vi "Leap Read.vi"(8 "error in (no error)":errorcluster, 11 "Leap Handle In":T14) -> (0 "error out":errorcluster, 2 "Frame":T1, 3 "Leap Handle Passthrough":T14, 5 "Leap Connected?":bool)   [LabVIEW 2011, in "LVH-Leap.lvlib"]
doc: "<b>Leap Read</b> requests and parses a <b>Frame</b> of data from the Leap Motion Controller. All the data associated with the Frame is organized into a LabVIEW cluster for accessibility.\n\nSpecifics about the data in the Frame cluster can be found by going to <b>Help » Leap Motion Controller Help</b> inside of LabVIEW"
uses:
  LVH-Leap.lvlib
  Private/Type Defs/Leap Handle.ctl
  C:/github/labviewhacker/LVH-Leap/LabVIEW/vi.lib/LabVIEW Hacker/Leap/Private/Libs/LeapCSharp.NET3.5.dll
  Private/Libs/LeapCSharp.NET3.5.dll
  Private/Type Defs/Frame.ctl
  Private/Type Defs/Hand.ctl
  Private/Type Defs/Vector.ctl
  Private/Type Defs/Pointable.ctl
  Private/Type Defs/Pointable Type.ctl
  Private/Type Defs/Pointable Zone.ctl
  Private/Type Defs/Gesture Key Tap.ctl
  Private/Type Defs/Gesture Common.ctl
  Private/Type Defs/Gesture Type.ctl
  Private/Type Defs/Gesture State.ctl
  Private/Type Defs/Gesture Screen Tap.ctl
  Private/Type Defs/Gesture Circle.ctl
  Private/Type Defs/Gesture Swipe.ctl
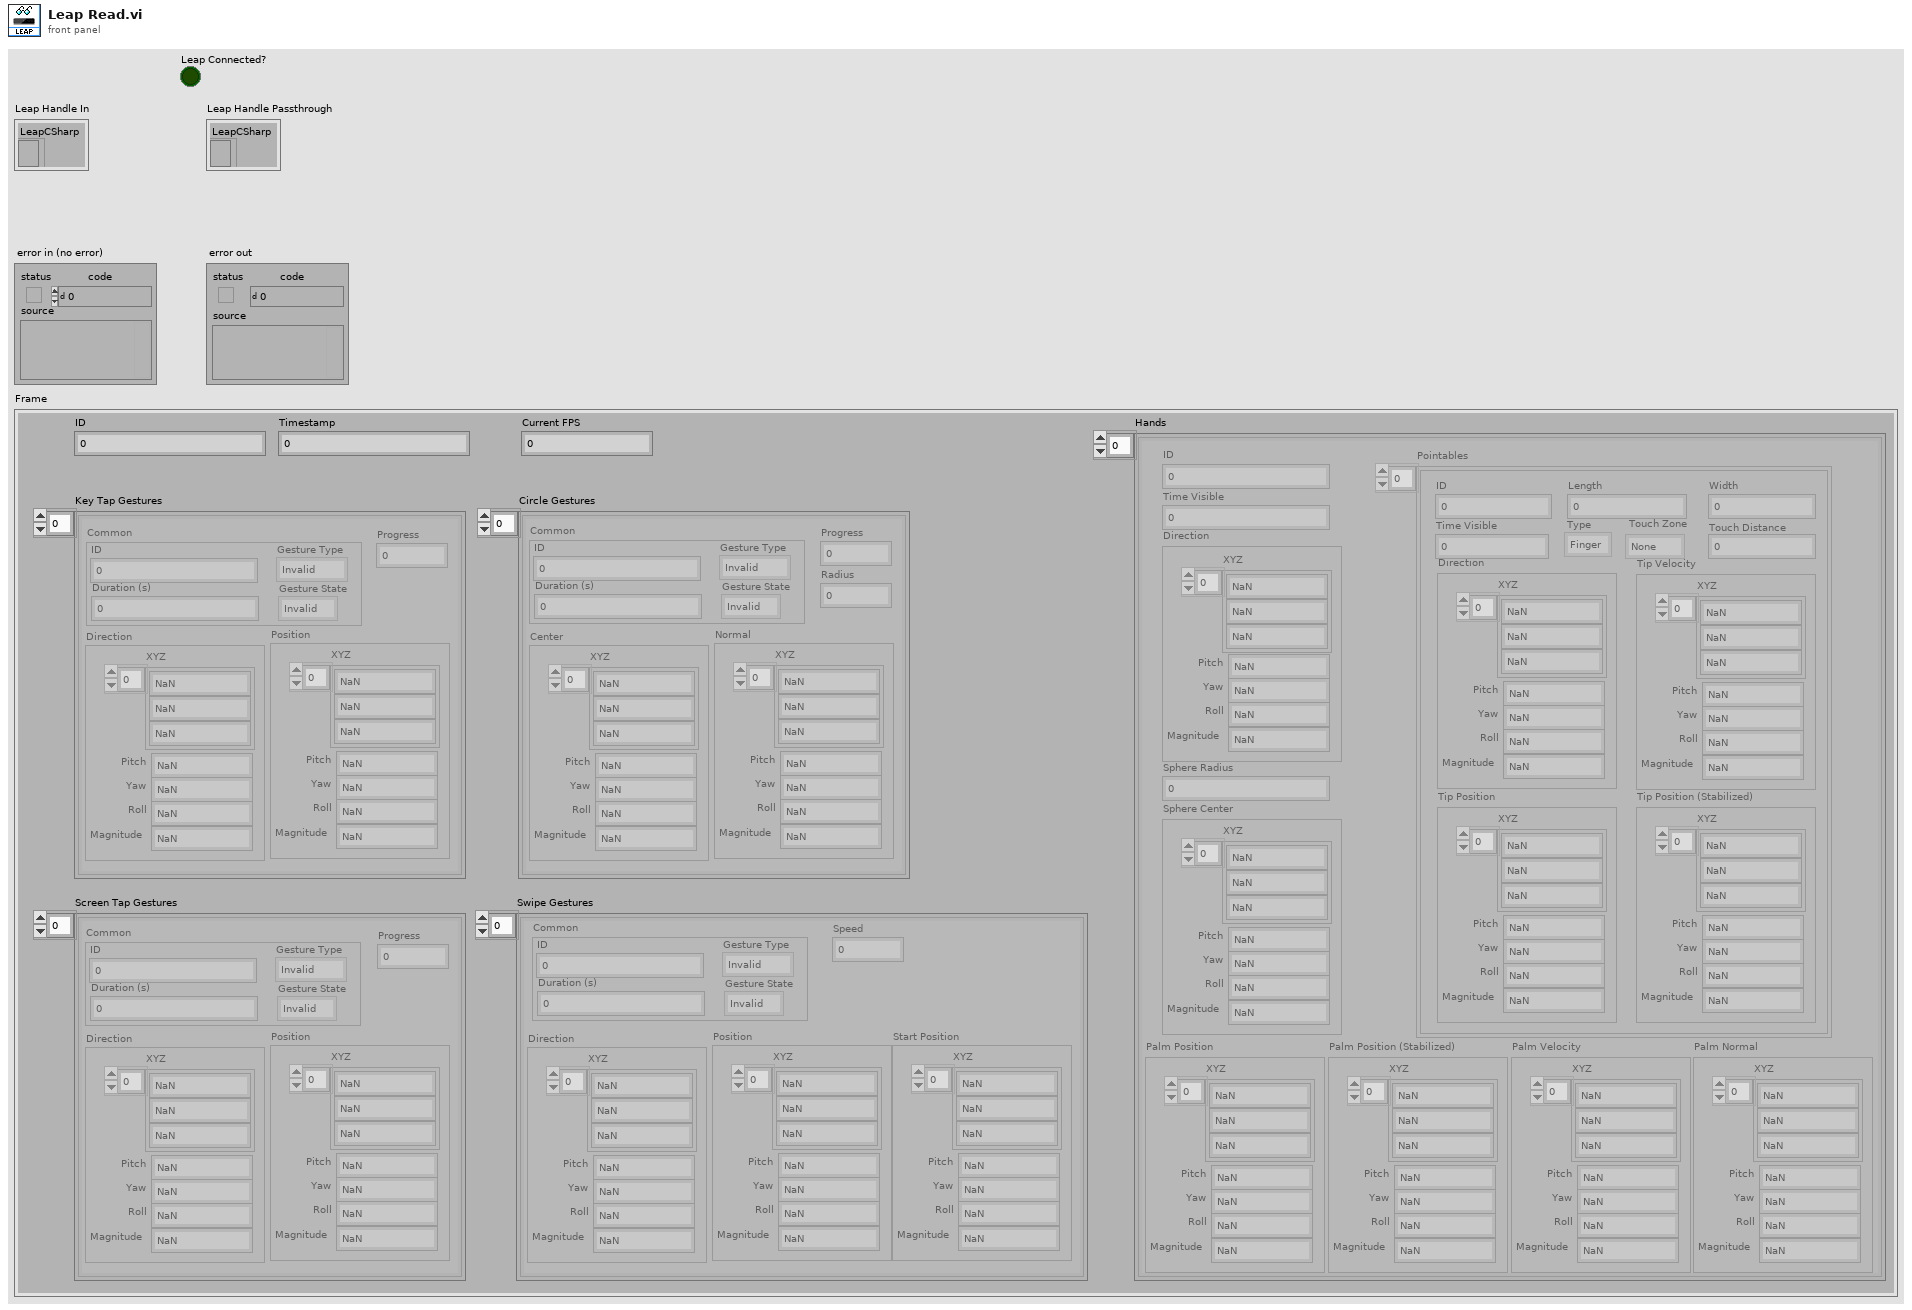
[diagram p1: front panel]
types:
  T1 = typedef "LVH-Leap.lvlib/Frame.ctl" = cluster{"ID":i64, "Timestamp":i64, "Hands":T2[], "Key Tap Gestures":T7[], "Screen Tap Gestures":T11[], "Circle Gestures":T12[], "Swipe Gestures":T13[], "Current FPS":dbl}
  T2 = typedef "LVH-Leap.lvlib/Hand.ctl" = cluster{"ID":i32, "Time Visible":sgl, "Direction":T3, "Palm Position":T3, "Palm Position (Stabilized)":T3, "Palm Velocity":T3, "Palm Normal":T3, "Pointables":T4[], "Sphere Radius":sgl, "Sphere Center":T3}
  T3 = typedef "LVH-Leap.lvlib/Vector.ctl" = cluster{"Pitch":sgl, "Yaw":sgl, "Roll":sgl, "Magnitude":sgl, "XYZ":sgl[]}
  T4 = typedef "LVH-Leap.lvlib/Pointable.ctl" = cluster{"ID":i32, "Length":dbl, "Width":dbl, "Time Visible":dbl, "Type":T5, "Direction":T3, "Tip Velocity":T3, "Tip Position":T3, "Tip Position (Stabilized)":T3, "Touch Zone":T6, "Touch Distance":dbl}
  T5 = typedef "LVH-Leap.lvlib/Pointable Type.ctl" = enum16{"Finger", "Tool"}
  T6 = typedef "LVH-Leap.lvlib/Pointable Zone.ctl" = enum16{"None", "Hovering", "Touching"}
  T7 = typedef "LVH-Leap.lvlib/Gesture Key Tap.ctl" = cluster{"Common":T8, "Direction":T3, "Position":T3, "Progress":dbl}
  T8 = typedef "LVH-Leap.lvlib/Gesture Common.ctl" = cluster{"ID":i32, "Duration (s)":dbl, "Gesture Type":T9, "Gesture State":T10}
  T9 = typedef "LVH-Leap.lvlib/Gesture Type.ctl" = enum16{"Invalid", "Swipe", "Circle", "Screen Tap", "Key Tap"}
  T10 = typedef "LVH-Leap.lvlib/Gesture State.ctl" = enum16{"Invalid", "Start", "Update", "Stop"}
  T11 = typedef "LVH-Leap.lvlib/Gesture Screen Tap.ctl" = cluster{"Common":T8, "Direction":T3, "Position":T3, "Progress":dbl}
  T12 = typedef "LVH-Leap.lvlib/Gesture Circle.ctl" = cluster{"Common":T8, "Center":T3, "Normal":T3, "Progress":dbl, "Radius":dbl}
  T13 = typedef "LVH-Leap.lvlib/Gesture Swipe.ctl" = cluster{"Common":T8, "Direction":T3, "Position":T3, "Start Position":T3, "Speed":dbl}
  T14 = typedef "LVH-Leap.lvlib/Leap Handle.ctl" = cluster{"LeapCSharp":refnum<k24>}
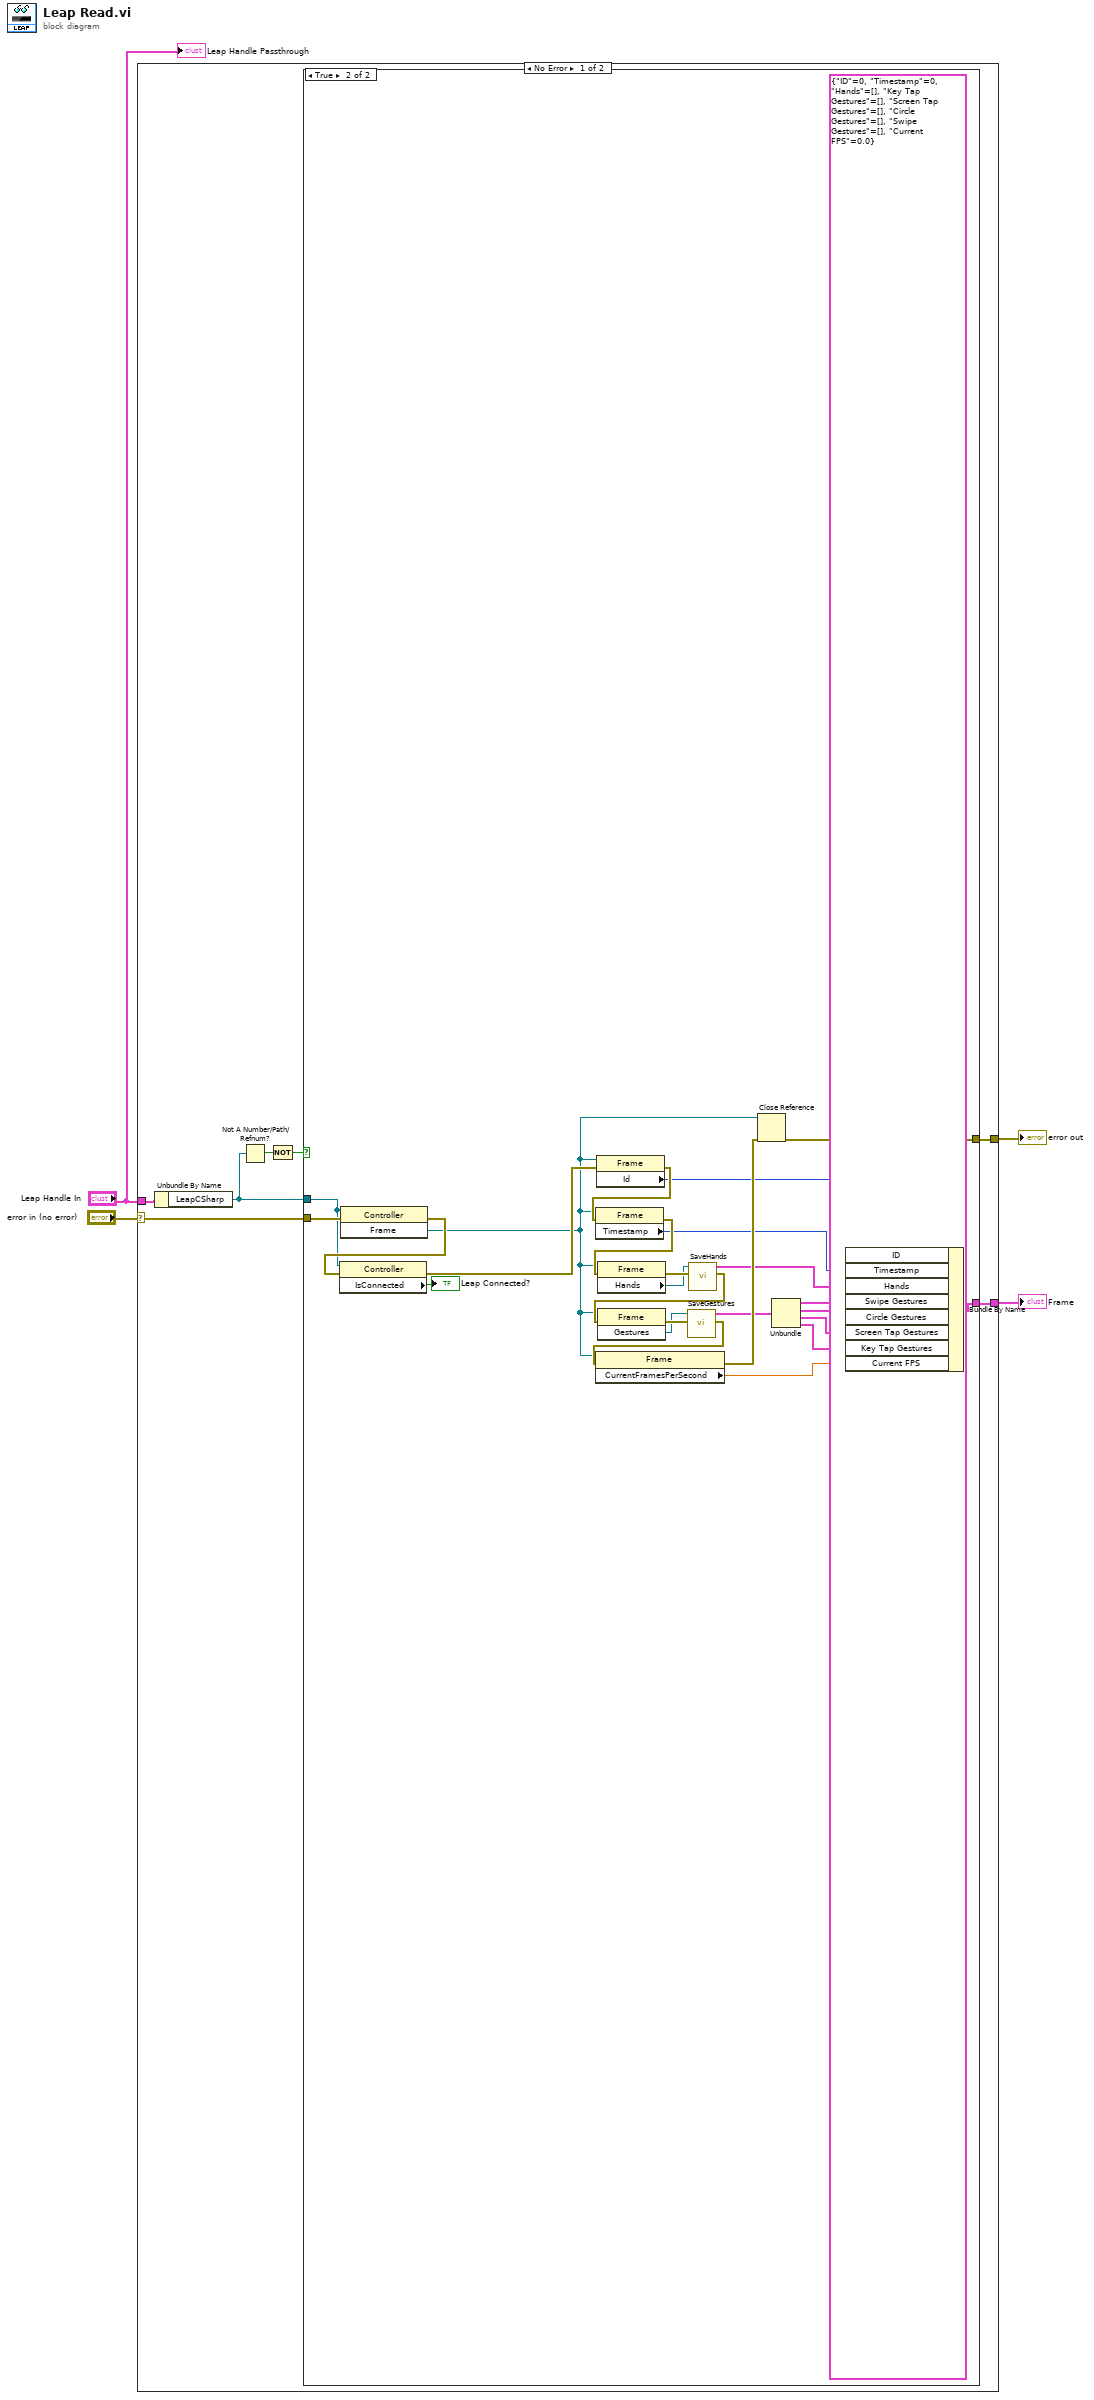
[diagram p0: block diagram]
diagram:
  n1 = case shown="No Error" "error in (no error)" {
    selector: "error in (no error)" -> [w9 w40]
    tunnel: "Leap Handle In" -> [w11 _]
    tunnel: [w10 _] -> w1
    tunnel: [w8 w40] -> w2
    frame No Error {
      n2 = Unbundle By Name(w11) -> ("LeapCSharp"=w5:refnum<k24>)
      n3 = Not A Number/Path/Refnum?(number/path/refnum=w5) -> (NaN/Path/Refnum?=w7:bool)
      n4 = Not(x=w7) -> (.not. x?=w6:bool)
      n5 = case shown="True" w6 {
        tunnel: [_ w30] -> w10
        tunnel: w5 -> [_ w27]
        tunnel: w9 -> [w12 w37]
        tunnel: [w12 w25] -> w8
        frame False {
        }
        frame True {
          n6 = invoke class="Controller" method="Frame"(reference=w27, error in=w37) -> (error out=w31:errorcluster, "Frame"=w14:refnum<k24>)  [unwired: 1 in, 1 out]
          n7 = property class="Controller"(reference=w27, error in=w31) -> (error out=w32:errorcluster, "IsConnected"=→"Leap Connected?":bool)  [unwired: 1 out]
          n8 = property class="Frame"(reference=w14, error in=w32) -> (error out=w33:errorcluster, "Id"=w16:i64)  [unwired: 1 out]
          n9 = property class="Frame"(reference=w14, error in=w33) -> (error out=w34:errorcluster, "Timestamp"=w17:i64)  [unwired: 1 out]
          n10 = property class="Frame"(reference=w14, error in=w34) -> (error out=w35:errorcluster, "Hands"=w29:refnum<k24>)  [unwired: 1 out]
          n11 = call "SaveHands.vi"("error in (no error)"=w35, ".NET Refnum in"=w29) -> ("error out"=w15:errorcluster, "Hands"=w18:T2[])  [unwired: 8 in]
          n12 = invoke class="Frame" method="Gestures"(reference=w14, error in=w15) -> (error out=w36:errorcluster, "Gestures"=w24:refnum<k24>)  [unwired: 1 in, 1 out]
          n13 = call "SaveGestures.vi"("error in (no error)"=w36, ".NET Refnum in"=w24) -> ("error out"=w39:errorcluster, "All Gestures"=w23:cluster{T13[], T12[], T11[], T7[]})  [unwired: 8 in]
          n14 = property class="Frame"(reference=w14, error in=w39) -> (error out=w38:errorcluster, "CurrentFramesPerSecond"=w13:sgl)  [unwired: 1 out]
          n15 = Close Reference(reference=w14, error in (no error)=w38) -> (error out=w25:errorcluster)
          n16 = Unbundle(w23) -> (w22:T13[], w21:T12[], w20:T11[], w19:T7[])
          n17 = Bundle By Name(cluster=T1 {"ID"=0, "Timestamp"=0, "Hands"=[], "Key Tap Gestures"=[], "Screen Tap Gestures"=[], "Circle Gestures"=[], "Swipe Gestures"=[], "Current FPS"=0.0} ("Frame"), "ID"=w16, "Timestamp"=w17, "Hands"=w18, "Swipe Gestures"=w22, "Circle Gestures"=w21, "Screen Tap Gestures"=w20, "Key Tap Gestures"=w19, "Current FPS"=w13) -> (w30:T1)
        }
      }
    }
    frame Error {
    }
  }
  "error out" <- w2
  "Frame" <- w1
  "Leap Handle Passthrough" <- "Leap Handle In"
